vi "Elog_.vi"() -> ()   [LabVIEW 2015]
uses:
  <vilib>/Platform/TimedLoop/XDataNode/timing_clust.ctl
  <vilib>/Platform/TimedLoop/XDataNode/nitl_modes.ctl
  <vilib>/Platform/TimedLoop/XDataNode/wakeup.ctl
  <userlib>/caLab/Private/Get_PV-1D.vi
  <vilib>/platform/TimedLoop/XDataNode/XDataNode.xnode
  <vilib>/Platform/TimedLoop/XDataNode/XDNodeRunTimeDep.lvlib
panel:
  out "spreadsheet string 3":string
  out "concatenated string 6":string
  out "standard error 3":string
  out "standard output 3":string
  in  "OK Button":bool
  in  "stop 2":bool
  in  "ELOG":string
  out "PV Names (dup)":string[](array[string])
  out "PV2ELOG":string
  # "Set a folder to watch using the\nPath control. You can also\nset a filter for a certain type\nof file to watch for (such as\n*.bmp). Then run the\nexample. Whenever you create\na new file in that directory that\nmatches the filter, New File Name\nwill update to let you know the\nnew file name."
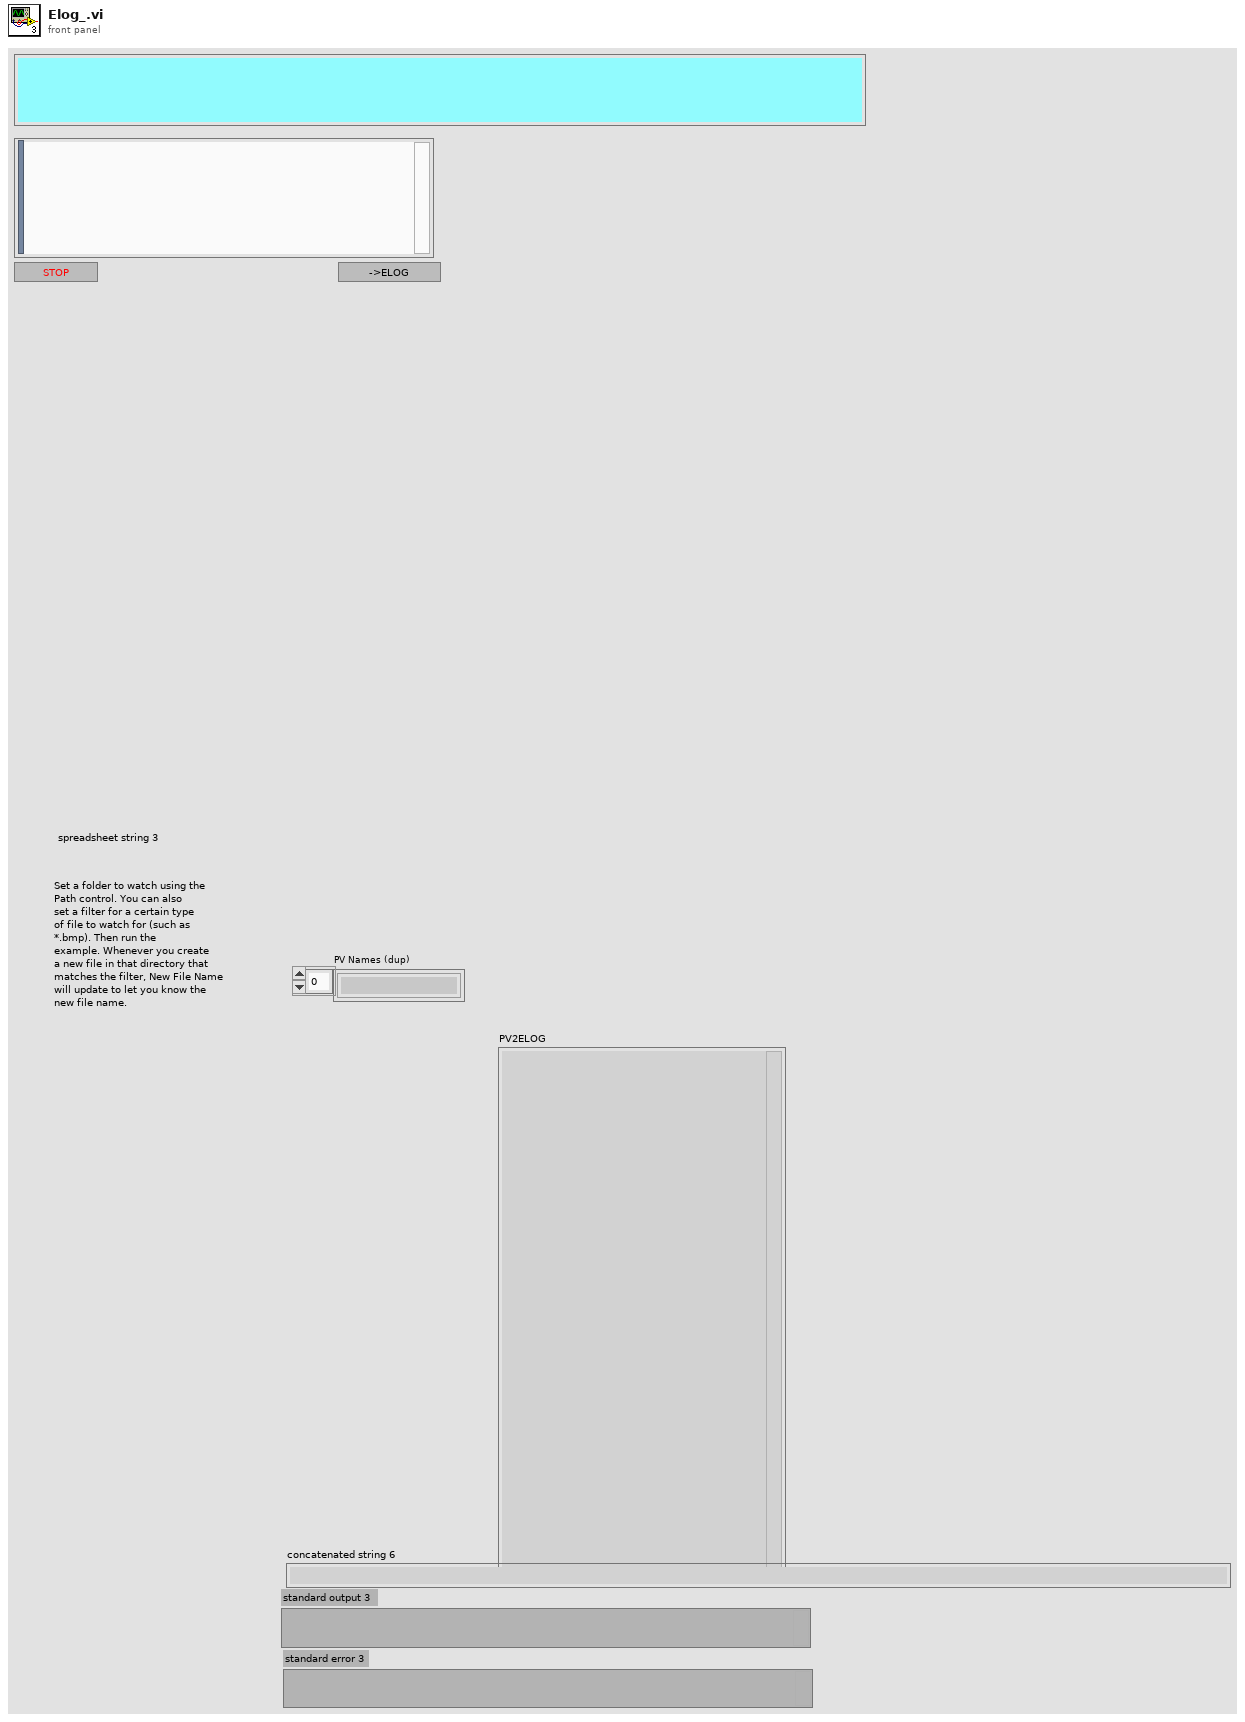
[diagram p1: front panel]
types:
  T1 = typedef "XDNodeRunTimeDep.lvlib/timing_clust.ctl" = cluster{"Expected End [f-1]":u64, "Actual End [f-1]":u64, "Finished Late? [f-1]":bool, "Expected End [i-1]":u64, "Actual End [i-1]":u64, "Finished Late? [i-1]":bool, "Expected Start [i]":u64, "Actual Start [i]":u64, "Expected Start [f]":u64, "Actual Start [f]":u64, "Source Name":string, "Structure Name":string, "Period":i64, "Deadline":i64, "Offset":i64, "Start":i64, "Priority":i32, "Timeout":i32, "Mode":T2, "Wakeup Reason":T3, "Error":errorcluster, "Source Type":string, "Secondary Source Type":string, "Global End Time":u64, "Global Start Time":u64, "Frame Duration":u64, "Iteration Duration":u64, "Assigned CPU":i32, "I/O Scan Engine Mode":u32}
  T2 = typedef "XDNodeRunTimeDep.lvlib/nitl_modes.ctl" = enum32{"No Change", "Process missed periods, maintain original phase", "Discard missed periods, maintain original phase", "Process missed periods, ignore original phase", "Discard missed periods, ignore original phase"}
  T3 = typedef "XDNodeRunTimeDep.lvlib/wakeup.ctl" = enum32{"Normal", "Aborted", "Asynchronous wakeup", "Timing source error", "Timed loop error", "Timeout"}
  T4 = enum16{"open", "replace", "create", "open or create", "replace or create", "replace or create with confirmation"}
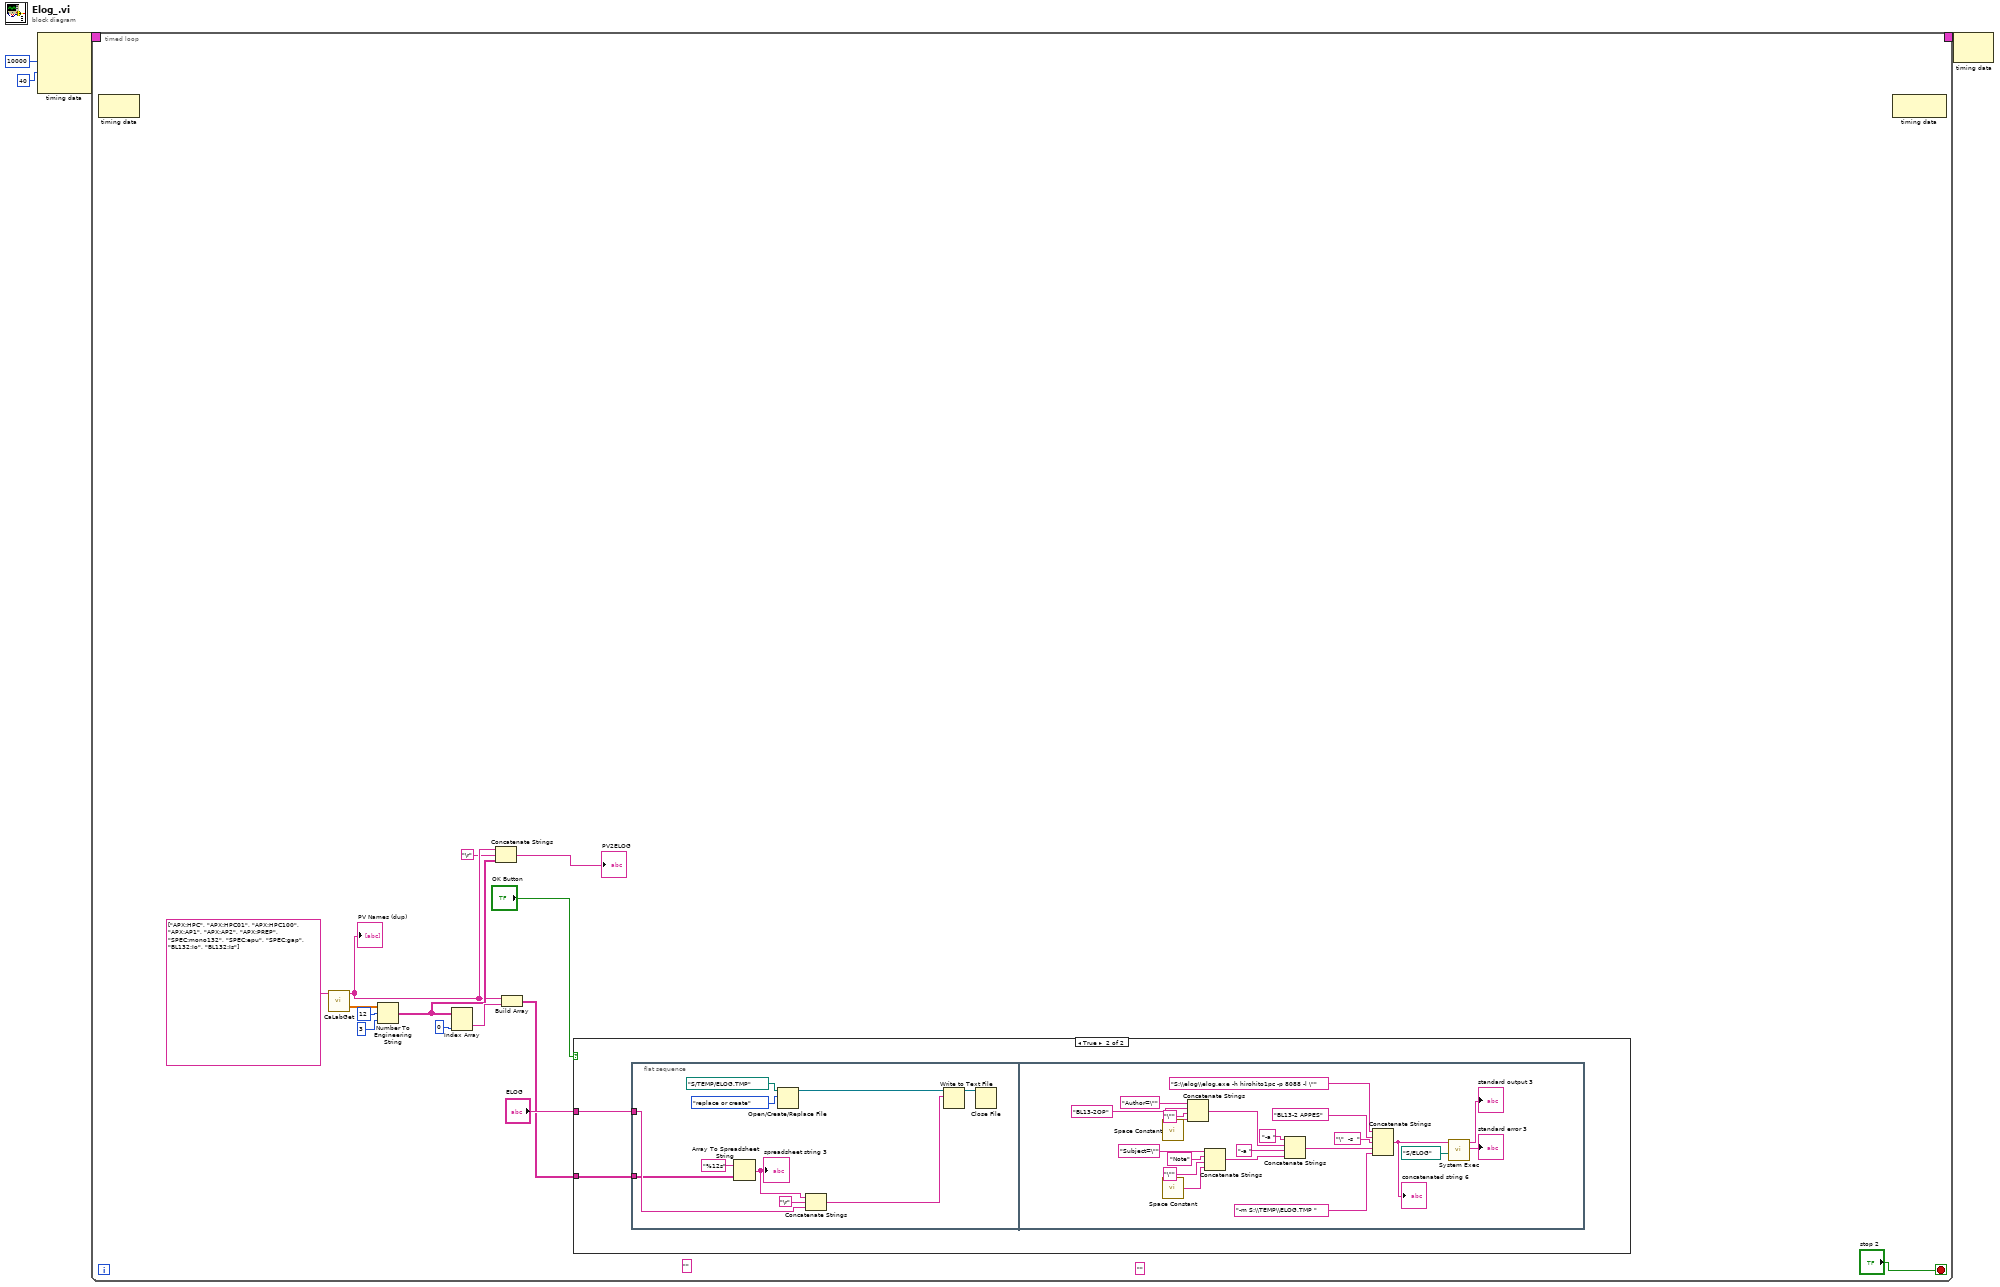
[diagram p0: block diagram]
diagram:
  n1 = node-c288(i64 10000 ("Period"), 40 ("Priority")) -> (w4:T1)  [unwired: 2 in]
  n2 = timed-loop {
    timing: w4 -> [_]
    timing-out: [_] -> w3
    stop <- "stop 2" stop-if-true
    (unwired) "" ("string")
    (unwired) "" ("string")
    n3 = node-c288() -> ()  [unwired: 1 in, 1 out]
    n4 = call-poly <userlib>:"CaLabGet.vi"("PV Names"=string[] ["APX:HPC", "APX:HPC01", "APX:HPC100", "APX:AP1", "APX:AP2", "APX:PREP", "SPEC:mono132", "SPEC:epu", "SPEC:gap", "BL132:Io", "BL132:Is"]) -> ("PV Names (dup)"=w12:string[], "Value Array (number)"=w10:dbl[][])  [unwired: 8 in, 5 out]
    "PV Names (dup)" <- w12
    n5 = Number To Engineering String(2:i16 3 ("precision (6)"), 3:i16 12 ("width (-)"), 4:w10) -> (0:w14:string[][])  [unwired: 1 in]
    n6 = Index Array(array=w14, index (col)=0) -> (element=w15:string[])  [unwired: 1 in]
    n7 = Concatenate Strings(w12, "\r", w14) -> (→"PV2ELOG":string)
    n8 = Build Array(w12, w15) -> (w5:string[][])
    n9 = case shown="True" "OK Button" {
      tunnel: "ELOG" -> [_ w20]
      tunnel: w5 -> [_ w19]
      frame False {
      }
      frame True {
        n10 = flat-sequence {
          tunnel: w20 -> [w22]
          tunnel: w19 -> [w21]
          frame #0 {
            n11 = Array To Spreadsheet String(array=w21, 3:"%12s" ("format string")) -> (spreadsheet string=w24:string)  [unwired: 1 in]
            "spreadsheet string 3" <- w24
            n12 = Open/Create/Replace File(file path (use dialog)=path "S:/TEMP/ELOG.TMP", operation (0:open)=T4."replace or create") -> (refnum out=w30:refnum<file>)  [unwired: 4 in, 2 out]
            n13 = Concatenate Strings(w24, "\r", w22) -> (w23:string)
            n14 = Write to Text File(file (use dialog)=w30, text=w23) -> (refnum out=w29:refnum<file>)  [unwired: 2 in, 2 out]
            n15 = Close File(refnum=w29) -> ()  [unwired: 1 in, 2 out]
          }
          frame #1 {
            n16 = call <vilib>:"Space Constant.vi"() -> ("String"=w37:string)
            n17 = call <vilib>:"Space Constant.vi"() -> ("String"=w38:string)
            n18 = Concatenate Strings("Author=\"" ("string"), "BL13-2OP", "\"" ("string"), w37) -> (w35:string)
            n19 = Concatenate Strings("Subject=\"" ("string"), "Note" ("string"), "\"" ("string"), w38) -> (w33:string)
            n20 = Concatenate Strings("-a ", w35, "-a " ("string"), w33) -> (w34:string)
            n21 = Concatenate Strings("S:\\elog\\elog.exe -h hirohito1pc -p 8088 -l \"" ("command line"), "BL13-2 APPES", "\"  -s  " ("command line"), w34, "-m S:\\TEMP\\ELOG.TMP " ("string")) -> (w46:string)
            "concatenated string 6" <- w46
            n22 = call <vilib>:"System Exec.vi"("working directory"=path "S:/ELOG", "command line"=w46) -> ("standard error"=→"standard error 3":string, "standard output"=→"standard output 3":string)  [unwired: 6 in, 2 out]
          }
        }
      }
    }
    n23 = node-c288() -> ()  [unwired: 1 in, 1 out]
  }
  n24 = node-c288(w3) -> ()  [unwired: 1 out]
